vi "DrawEllipseArcLength.vi"(8 "b":dbl, 9 "a":dbl, 10 "t":dbl, 11 "Dt":dbl) -> (1 "Ds'":dbl format="%.2f", 3 "Ds":dbl format="%.2f")   [LabVIEW 2017]
uses:
  <vilib>/gmath/SpecialFunctions.llb/Incomplete Elliptic Integral E.vi
  <vilib>/gmath/NI_Gmath.lvlib
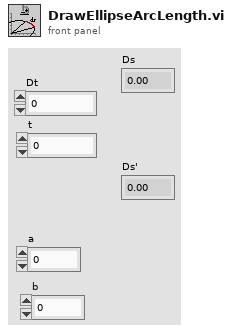
[diagram p1: front panel]
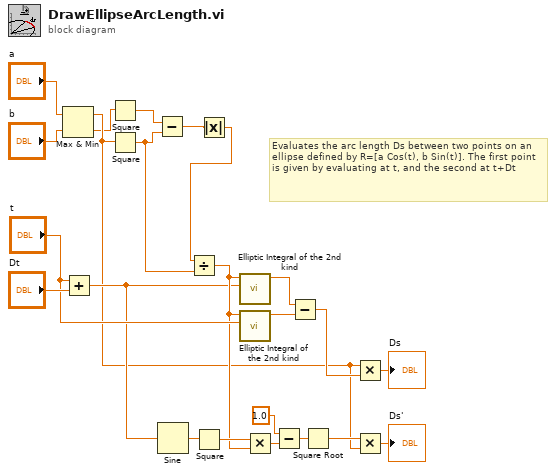
[diagram p0: block diagram]
diagram:
  # "Evaluates the arc length Ds between two points on an ellipse defined by R=[a Cos(t), b Sin(t)]. The first point is given by evaluating at t, and the second at t+Dt"
  n1 = Max & Min(x="a", y="b") -> (max(x,y)=w4:dbl, min(x,y)=w3:dbl)
  n2 = Add(x="t", y="Dt") -> (x+y=w9:dbl)
  n3 = Square(x=w3) -> (x^2=w8:dbl)
  n4 = Square(x=w4) -> (x^2=w7:dbl)
  n5 = Subtract(x=w8, y=w7) -> (x-y=w6:dbl)
  n6 = Sine(x=w9) -> (sin(x)=w16:dbl)
  n7 = Square(x=w16) -> (x^2=w17:dbl)
  n8 = Absolute Value(x=w6) -> (abs(x)=w5:dbl)
  n9 = Divide(x=w5, y=w7) -> (x/y=w13:dbl)
  n10 = call-poly <vilib>:"Elliptic Integral of the 2nd kind.vi"("a"=w9, "k"=w13) -> ("E(k, a)"=w12:dbl)  [unwired: 9 in]
  n11 = call-poly <vilib>:"Elliptic Integral of the 2nd kind.vi"("a"="t", "k"=w13) -> ("E(k, a)"=w11:dbl)  [unwired: 9 in]
  n12 = Multiply(x=w17, y=w13) -> (x*y=w21:dbl)
  n13 = Subtract(x=1.0 ("y"), y=w21) -> (x-y=w20:dbl)
  n14 = Subtract(x=w12, y=w11) -> (x-y=w10:dbl)
  n15 = Square Root(x=w20) -> (sqrt(x)=w19:dbl)
  n16 = Multiply(x=w4, y=w10) -> (x*y=→"Ds":dbl)
  n17 = Multiply(x=w19, y=w4) -> (x*y=→"Ds'":dbl)
